vi "PythonWriteRead.vi"(0 "connection in":refnum<k5>, 5 "string in":string, 7 "error in":errorcluster, 9 "timeout in":i32=-1, 11 "run_tcp in":bool) -> (4 "connection out":refnum<k5>, 6 "string out":string, 8 "error out":errorcluster, 10 "timeout out":i32=-1, 15 "run_tcp out":bool)   [LabVIEW 2014]
panel:
  out "read bytes":i32
  out "read header size":u32
  out "written bytes":i32
  out "write header written size":i32
  out "write payload size hex":string
  out "write payload size":i32
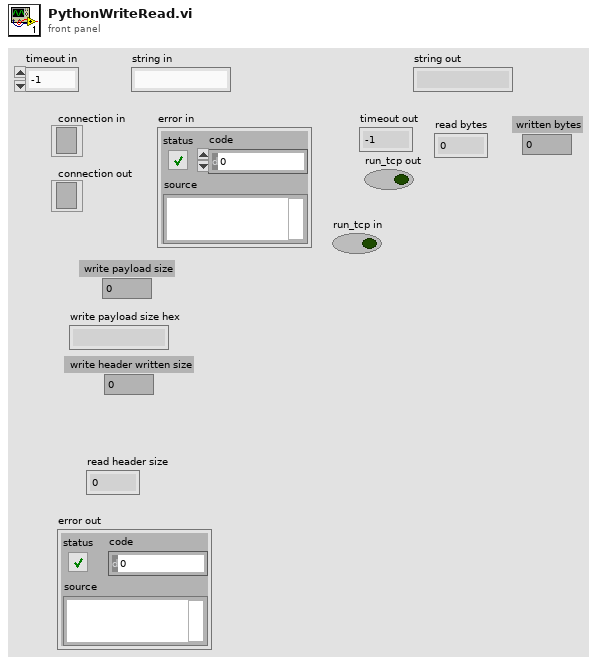
[diagram p1: front panel]
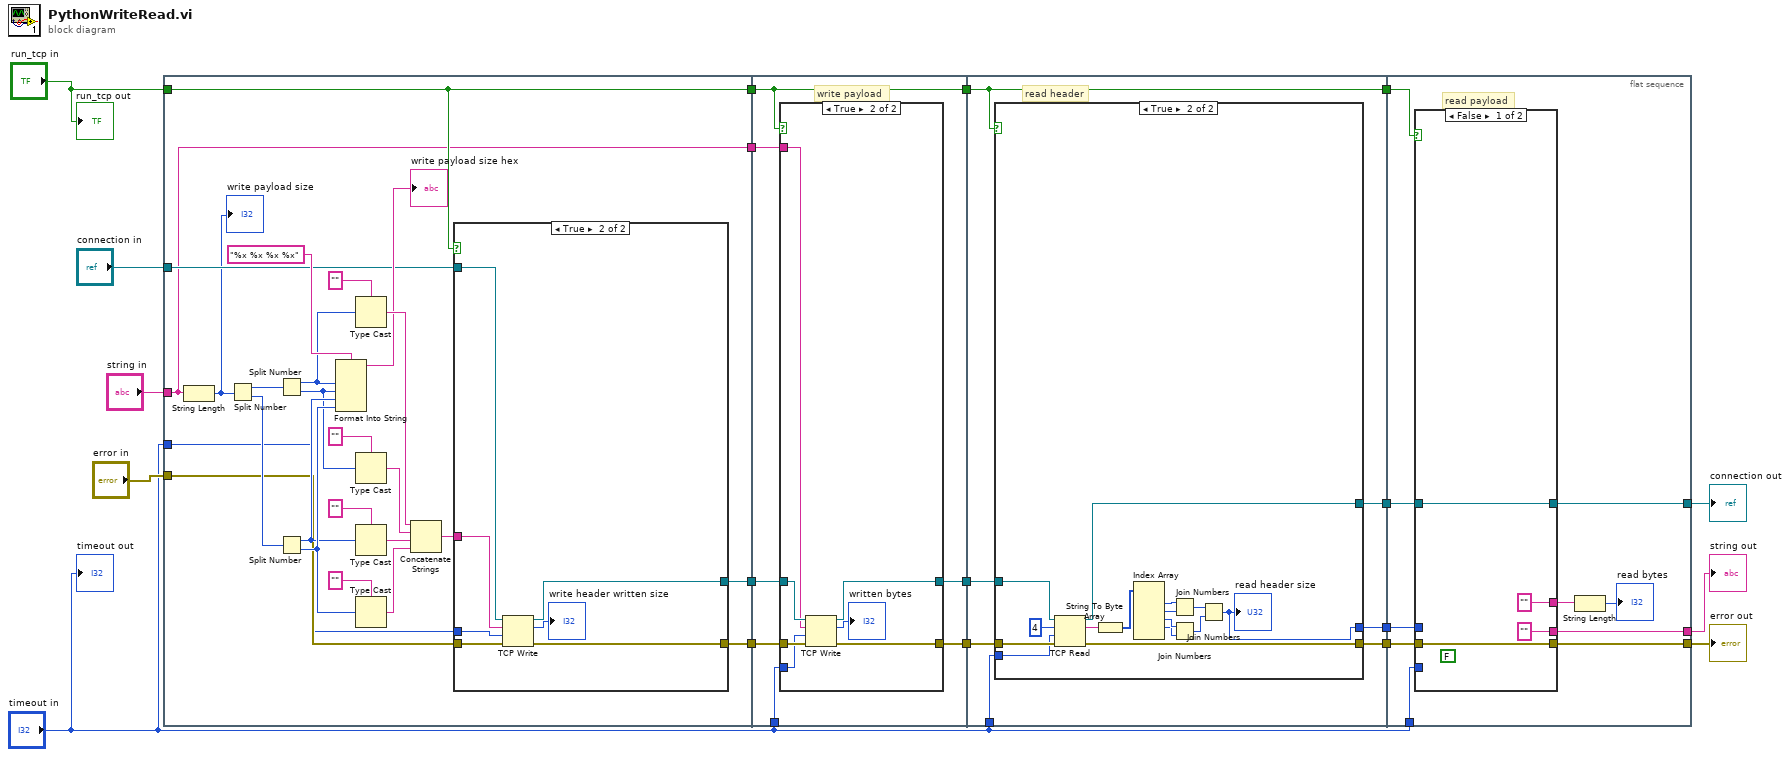
[diagram p0: block diagram]
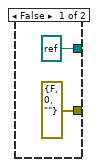
[diagram p2: hidden frame]
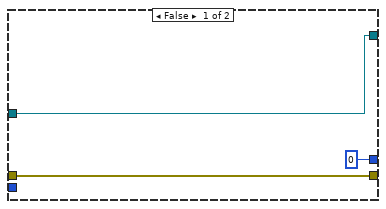
[diagram p4: hidden frame]
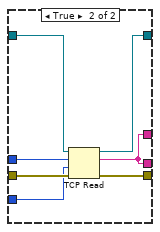
[diagram p5: hidden frame]
diagram:
  n1 = flat-sequence {
    tunnel: [w27] -> w19
    tunnel: [w20] -> w18
    tunnel: [w26] -> w17
    tunnel: "error in" -> [w25]
    tunnel: "connection in" -> [w24]
    tunnel: "run_tcp in" -> [w23]
    tunnel: [w23] -> w7
    tunnel: "timeout in" -> [w21]
    tunnel: "string in" -> [w20]
    tunnel: w19 -> [w60]
    tunnel: w18 -> [w59]
    tunnel: w17 -> [w58]
    tunnel: [w57] -> w16
    tunnel: [w56] -> w15
    tunnel: w7 -> [w55]
    tunnel: [w55] -> w6
    tunnel: "timeout in" -> [w54]
    tunnel: w16 -> [w76]
    tunnel: w15 -> [w75]
    tunnel: [w74] -> w14
    tunnel: [w73] -> w13
    tunnel: [w72] -> w12
    tunnel: w6 -> [w71]
    tunnel: [w71] -> w5
    tunnel: "timeout in" -> [w70]
    tunnel: w14 -> [w104]
    tunnel: w13 -> [w103]
    tunnel: w12 -> [w102]
    tunnel: w5 -> [w99]
    tunnel: "timeout in" -> [w96]
    tunnel: [w101] -> w9
    tunnel: [w100] -> w8
    tunnel: [w95] -> w3
    frame #0 {
      n2 = String Length(string=w20) -> (length=w22:i32)
      "write payload size" <- w22
      n3 = Split Number(x=w22) -> (hi(x)=w35:u16, lo(x)=w36:u16)
      n4 = Split Number(x=w35) -> (hi(x)=w30:u8, lo(x)=w31:u8)
      n5 = Split Number(x=w36) -> (hi(x)=w32:u8, lo(x)=w33:u8)
      n6 = Format Into String(format string="%x %x %x %x" ("type"), w30, w31, w32, w33) -> (resulting string=→"write payload size hex":string)  [unwired: 2 in, 1 out]
      n7 = Type Cast(type="", x=w30) -> (*(type *) &x=w41:string)
      n8 = Type Cast(type="", x=w31) -> (*(type *) &x=w42:string)
      n9 = Type Cast(type="", x=w32) -> (*(type *) &x=w43:string)
      n10 = Type Cast(type="", x=w33) -> (*(type *) &x=w44:string)
      n11 = Concatenate Strings(w41, w42, w43, w44) -> (w28:string)
      n12 = case shown="True" w23 {
        tunnel: w28 -> [_ w53]
        tunnel: [refnum<k5> refnum ("connection ID") w51] -> w27
        tunnel: [errorcluster {"status"=FALSE, "code"=0, "source"=""} ("error out") w50] -> w26
        tunnel: w25 -> [_ w49]
        tunnel: w24 -> [_ w48]
        tunnel: w21 -> [_ w47]
        frame False {
        }
        frame True {
          n13 = TCP Write(connection ID=w48, data in=w53, error in (no error)=w49, 9:w47) -> (connection ID out=w51:refnum<k5>, bytes written=→"write header written size":i32, error out=w50:errorcluster)
        }
      }
    }
    frame #1 {
      # "write payload"
      n14 = case shown="True" w55 {
        tunnel: w60 -> [w61 w68]
        tunnel: w59 -> [_ w67]
        tunnel: w58 -> [w62 w66]
        tunnel: [w61 w65] -> w57
        tunnel: [w62 w64] -> w56
        tunnel: w54 -> [_ w63]
        frame False {
        }
        frame True {
          n15 = TCP Write(connection ID=w68, data in=w67, error in (no error)=w66, 9:w63) -> (connection ID out=w65:refnum<k5>, bytes written=→"written bytes":i32, error out=w64:errorcluster)
        }
      }
    }
    frame #2 {
      # "read header"
      n16 = case shown="True" w71 {
        tunnel: w76 -> [w78 w94]
        tunnel: w75 -> [w77 w92]
        tunnel: [w78 w83] -> w74
        tunnel: [w77 w82] -> w73
        tunnel: [u32 0 w81] -> w72
        tunnel: w70 -> [_ w80]
        frame False {
        }
        frame True {
          n17 = TCP Read(connection ID=w94, bytes to read=4, error in (no error)=w92, 9:w80) -> (connection ID out=w83:refnum<k5>, data out=w91:string, error out=w82:errorcluster)  [unwired: 1 in]
          n18 = String To Byte Array(string=w91) -> (unsigned byte array=w90:u8[])
          n19 = Index Array(array=w90) -> (element #1=w89:u8, element #2=w88:u8, element #3=w87:u8, element #4=w86:u8)  [unwired: 5 in, 1 out]
          n20 = Join Numbers(hi=w89, lo=w88) -> ((hi.lo)=w85:u16)
          n21 = Join Numbers(hi=w87, lo=w86) -> ((hi.lo)=w84:u16)
          n22 = Join Numbers(hi=w85, lo=w84) -> ((hi.lo)=w81:u32)
          "read header size" <- w81
        }
      }
    }
    frame #3 {
      # "read payload"
      n23 = case shown="False" w99 {
        tunnel: w104 -> [w107 w115]
        tunnel: w103 -> [w108 w114]
        tunnel: w102 -> [_ w113]
        tunnel: [w107 w112] -> w101
        tunnel: [w108 w109] -> w100
        tunnel: ["" ("data out") w110] -> w98
        tunnel: w96 -> [_ w111]
        tunnel: ["" ("data out") w110] -> w95
        frame False {
          (unwired) FALSE ("stop")
        }
        frame True {
          n24 = TCP Read(connection ID=w115, bytes to read=w113, error in (no error)=w114, 9:w111) -> (connection ID out=w112:refnum<k5>, data out=w110:string, error out=w109:errorcluster)  [unwired: 1 in]
        }
      }
      n25 = String Length(string=w98) -> (length=→"read bytes":i32)
    }
  }
  "connection out" <- w9
  "error out" <- w8
  "string out" <- w3
  "timeout out" <- "timeout in"
  "run_tcp out" <- "run_tcp in"
